vi "Open OPC UA Connection.vi"(8 "error in (no error)":errorcluster, 10 "Connection Configuration":T2={"Client?"=FALSE, "Server Certificates"={"Relative Path?"=FALSE, "Certificate Paths"=[], "Certificate Names"=[]}, "Client Certificates"={"Relative Path?"=FALSE, "Certificate Paths"=[], "Certificate Names"=[]}, "Client Configuration"={"Server Endpoint URL"="", "Security Policy"={"Message Mode"=enum."None", "Security"=enum."Basic256"}, "Username/Password"={"Username"="", "Password"=""}}, "Server Configuration"={"Server Name"="", "TCP port (49580)"="49580", "Supported Security Policies"={"None"=TRUE, "Sign with Basic128Rsa125"=FALSE, "Sign and Encrypt with Basic128Rsa125"=FALSE, "Sign with Basic256"=FALSE, "Sign and Encrypt with Basic256"=FALSE}}}, 11 "OPC UA runtime in":refnum<class "OPC UA runtime.lvclass">) -> (0 "error out":errorcluster, 3 "OPC UA runtime out":refnum<class "OPC UA runtime.lvclass">)   [LabVIEW 2013, in "OPC UA runtime.lvclass"]
doc: "Opens connection to either an OPC UA Client or Server."
uses:
  OPC UA runtime.lvclass
  <vilib>/OPCUA/server/subVI/supported security policies.ctl
  OPC UA runtime.lvclass/OPC UA runtime.ctl
  <vilib>/opcua/NI OPC UA Server.lvlib
  <vilib>/opcua/NI OPC UA Client.lvlib
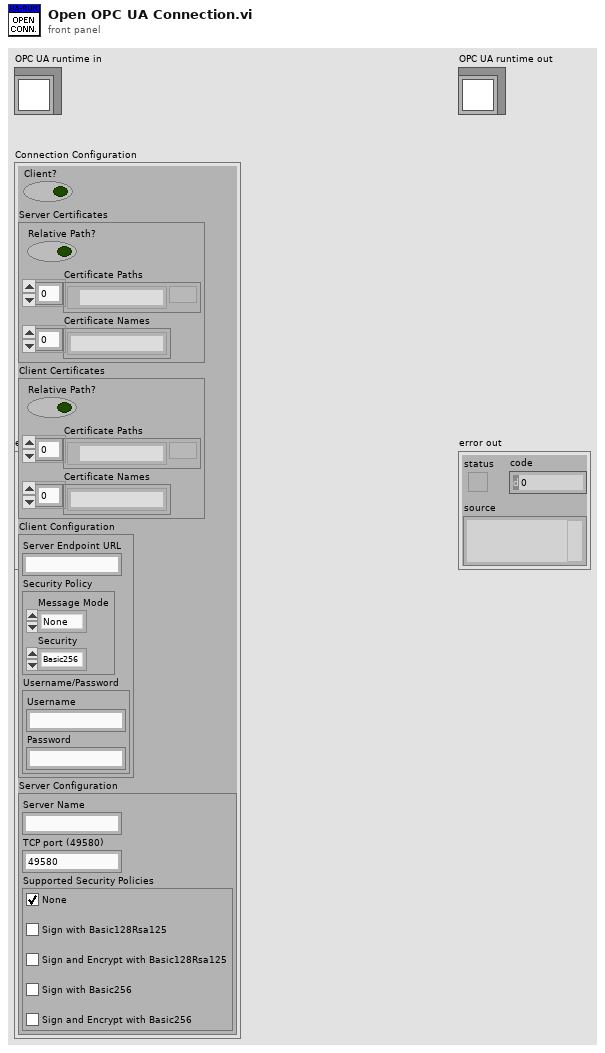
[diagram p1: front panel]
types:
  T1 = typedef "supported security policies.ctl" = cluster{"None":bool, "Sign with Basic128Rsa125":bool, "Sign and Encrypt with Basic128Rsa125":bool, "Sign with Basic256":bool, "Sign and Encrypt with Basic256":bool}
  T2 = cluster{"Client?":bool, "Server Certificates":cluster{"Relative Path?":bool, "Certificate Paths":path[], "Certificate Names":string[]}, "Client Certificates":cluster{"Relative Path?":bool, "Certificate Paths":path[], "Certificate Names":string[]}, "Client Configuration":cluster{"Server Endpoint URL":string, "Security Policy":cluster{"Message Mode":enum16{"None", "Sign", "Sign and Encrypt"}, "Security":enum16{"Basic256", "Basic128Rsa15"}}, "Username/Password":cluster{"Username":string, "Password":string}}, "Server Configuration":cluster{"Server Name":string, "TCP port (49580)":string, "Supported Security Policies":T1}}
  T3 = cluster{"Relative Path?":bool, "Certificate Paths":path[], "Certificate Names":string[]}
  T4 = cluster{"Message Mode":enum16{"None", "Sign", "Sign and Encrypt"}, "Security":enum16{"Basic256", "Basic128Rsa15"}}
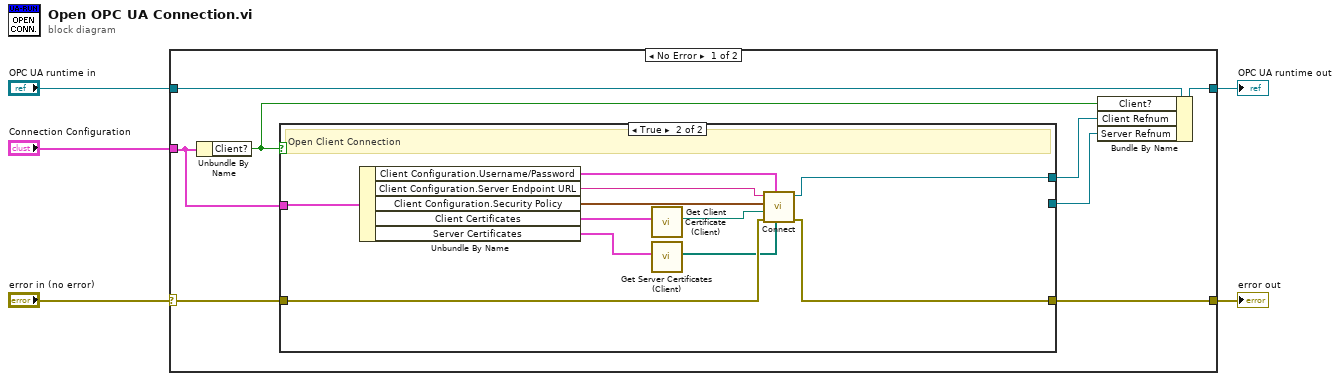
[diagram p0: block diagram]
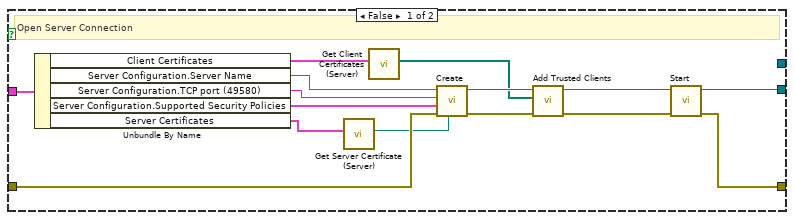
[diagram p2: hidden frame]
diagram:
  n1 = case shown="No Error" "error in (no error)" {
    selector: "error in (no error)" -> [w9 w41]
    tunnel: [w7 w41] -> w4
    tunnel: [w12 w40] -> w2
    tunnel: "OPC UA runtime in" -> [w13 w40]
    tunnel: "Connection Configuration" -> [w10 _]
    frame No Error {
      n2 = Unbundle By Name(w10) -> ("Client?"=w11:bool)
      n3 = case shown="True" w11 {
        tunnel: w10 -> [w28 w36]
        tunnel: w9 -> [w27 w39]
        tunnel: [w14 _] -> w8
        tunnel: [w15 w38] -> w7
        tunnel: [_ w37] -> w6
        frame False {
          # "Open Server Connection"
          n4 = Unbundle By Name(w28) -> ("Client Certificates"=w19:T3, "Server Configuration.Server Name"=w24:string, "Server Configuration.TCP port (49580)"=w25:string, "Server Configuration.Supported Security Policies"=w26:T1, "Server Certificates"=w23:T3)
          n5 = call "Get Server Certificate (Server).vi"("Server Certificates"=w23) -> ("server certificate file"=w22:path)  [unwired: 10 in]
          n6 = call "Get Client Certificates (Server).vi"("Client Certificates"=w19) -> ("trusted client certificates"=w18:path[])  [unwired: 10 in]
          n7 = call <vilib>:"Create.vi"("server certificate file"=w22, "error in (no error)"=w27, "supported security policies (None)"=w26, "TCP port (49580)"=w25, "OPC UA server name"=w24) -> ("error out"=w21:errorcluster, "OPC UA server refnum out"=w20:refnum<k21>)  [unwired: 4 in, 1 out]
          n8 = call <vilib>:"Add Trusted Clients.vi"("error in (no error)"=w21, "trusted client certificates"=w18, "OPC UA server refnum in"=w20) -> ("error out"=w17:errorcluster, "OPC UA server refnum out"=w16:refnum<k21>)  [unwired: 7 in]
          n9 = call <vilib>:"Start.vi"("error in (no error)"=w17, "OPC UA server refnum in"=w16) -> ("error out"=w15:errorcluster, "OPC UA server refnum out"=w14:refnum<k21>)  [unwired: 8 in]
        }
        frame True {
          # "Open Client Connection"
          n10 = Unbundle By Name(w36) -> ("Client Configuration.Username/Password"=w35:cluster{"Username":string, "Password":string}, "Client Configuration.Server Endpoint URL"=w34:string, "Client Configuration.Security Policy"=w33:T4, "Client Certificates"=w32:T3, "Server Certificates"=w30:T3)
          n11 = call "Get Client Certificate (Client).vi"("Client Certificates"=w32) -> ("client certificate file"=w31:path)  [unwired: 10 in]
          n12 = call "Get Server Certificates (Client).vi"("Server Certificates"=w30) -> ("trusted server certificates"=w29:path[])  [unwired: 10 in]
          n13 = call <vilib>:"Connect.vi"("trusted server certificates"=w29, "username/password"=w35, "error in (no error)"=w39, "client certificate file"=w31, "security policy"=w33, "server endpoint URL"=w34) -> ("error out"=w38:errorcluster, "OPC UA client refnum out"=w37:refnum<k21>)  [unwired: 3 in, 1 out]
        }
      }
      n14 = Bundle By Name(cluster=w13, "Client?"=w11, "Client Refnum"=w6, "Server Refnum"=w8) -> (w12:refnum<class "OPC UA runtime.lvclass">)
    }
    frame Error {
    }
  }
  "error out" <- w4
  "OPC UA runtime out" <- w2
